vi "StageInit.vi"(0 "error in":errorcluster, 3 "Stage in":refnum<vi>, 4 "Name":string="scene") -> (1 "error out":errorcluster, 5 "Stage out":refnum<vi>)   [LabVIEW 2018]
uses:
  <vilib>/picture/3D Picture Control/Object/Create Object (name).vi
  <vilib>/picture/3D Picture Control/NI_3D Picture Control.lvlib
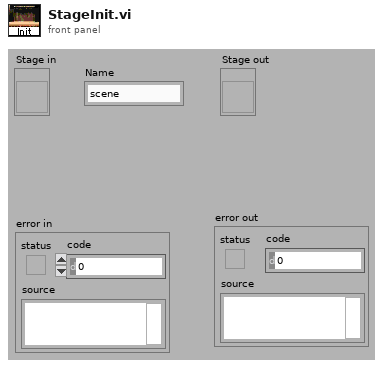
[diagram p1: front panel]
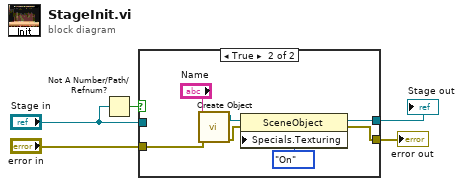
[diagram p0: block diagram]
diagram:
  n1 = Not A Number/Path/Refnum?(number/path/refnum="Stage in") -> (NaN/Path/Refnum?=w5:bool)
  n2 = case shown="True" w5 {
    tunnel: "error in" -> [w6 w13]
    tunnel: [w6 w8] -> w1
    tunnel: [w7 w10] -> w2
    tunnel: "Stage in" -> [w7 _]
    frame False {
    }
    frame True {
      n3 = call-poly <vilib>:"Create Object.vi"("error in (no error)"=w13, "Name"="Name") -> ("error out"=w9:errorcluster, "Scene:New Object"=w11:refnum<vi>)  [unwired: 8 in]
      n4 = property class="SceneObject"(reference=w11, error in=w9, "Specials.Texturing"=enum16{"Inherit Value", "Off", "On"}."On" ("Specials:Texturing")) -> (reference out=w10:refnum<vi>, error out=w8:errorcluster)
    }
  }
  "error out" <- w1
  "Stage out" <- w2
